vi "Wait Until Sees Fire.vi"(10 "Session In":T1, 11 "Sign File Path":path=path "C:/Users/EISD/Desktop/SVN Internal/Robot/Programming/Competition Code/cRIO Project/fire geo template super scale.png") -> (1 "Fire?":bool, 3 "Image":T2(plugin-control))   [LabVIEW 2013]
uses:
  <vilib>/userdefined/High Color/IMAQdx.ctl
  <vilib>/vision/driver/NI_Vision_Acquisition_Software.lvlib
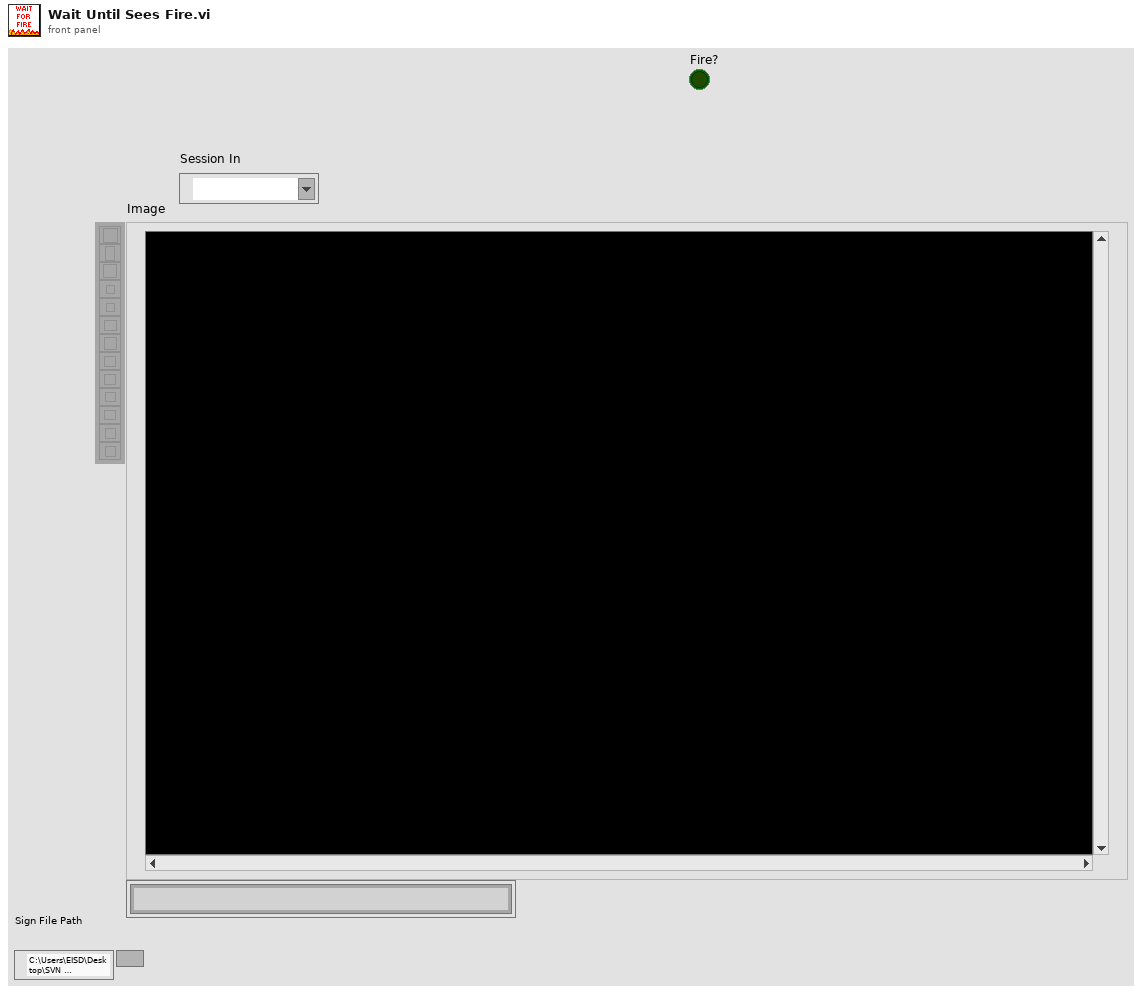
[diagram p1: front panel]
types:
  T1 = typedef "IMAQdx.ctl" = refnum<k21>
  T2 = typedef "IMAQ Image.ctl" = refnum<image>
  T3 = typedef "IMAQ GM Match Report.ctl" = cluster{"Position":cluster{"x":sgl, "y":sgl}, "Angle":sgl, "Scale":sgl, "Score":sgl, "Bounding Box":cluster{"x":sgl, "y":sgl}[], "Contrast Reversed":bool, "Occlusion %":sgl, "Template Target Curve Score":sgl, "Target Template Curve Score":sgl, "Correlation Score":sgl}
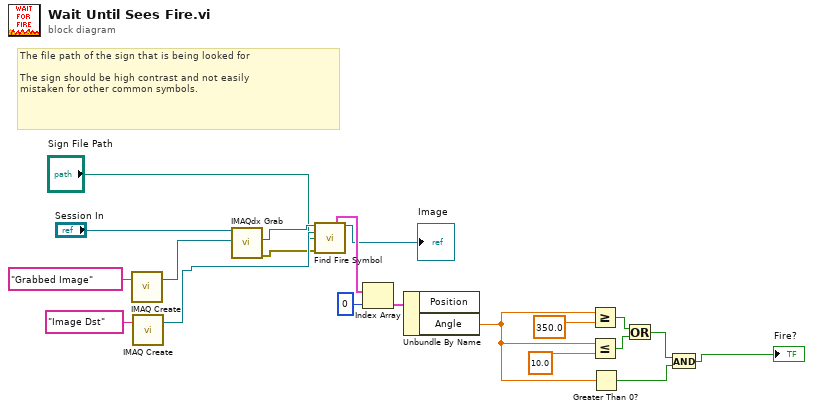
[diagram p0: block diagram]
diagram:
  # "The file path of the sign that is being looked for\n\nThe sign should be high contrast and not easily \nmistaken for other common symbols."
  n1 = call "IMAQ Create"("Image Name"="Grabbed Image") -> ("New Image"=w20:T2)  [unwired: 4 in, 1 out]
  n2 = call "IMAQ Create"("Image Name"="Image Dst") -> ("New Image"=w17:T2)  [unwired: 4 in, 1 out]
  n3 = call <vilib>:"IMAQdx Grab.vi"("Image In"=w20, "Session In"="Session In") -> ("error out"=w2:errorcluster, "Image Out"=w3:T2)  [unwired: 6 in, 2 out]
  n4 = call "Find Fire Symbol.vi"("Image In"=w3, "Image Dst"=w17, "Template File Path"="Sign File Path", "error in"=w2) -> ("Matches (Geometric Matching 1)"=w14:T3[], "Image Out"=→"Image":T2)  [unwired: 8 in, 2 out]
  n5 = Index Array(array=w14, index=0) -> (element=w12:T3)
  n6 = Unbundle By Name(w12) -> ("Angle"=w6:sgl)  [unwired: 1 out]
  n7 = Greater Or Equal?(x=w6, y=sgl 350.0) -> (x >= y?=w8:bool)
  n8 = Less Or Equal?(x=w6, y=sgl 10.0) -> (x <= y?=w9:bool)
  n9 = Greater Than 0?(x=w6) -> (x > 0?=w4:bool)
  n10 = Or(x=w8, y=w9) -> (x .or. y?=w5:bool)
  n11 = And(x=w5, y=w4) -> (x .and. y?=→"Fire?":bool)
